vi "RLSET.vi"(8 "错误输入（无错误）":errorcluster, 9 "BIT_L":string, 10 "BIT_H":string) -> (0 "error out":errorcluster caption="错误输出")   [LabVIEW 2018]
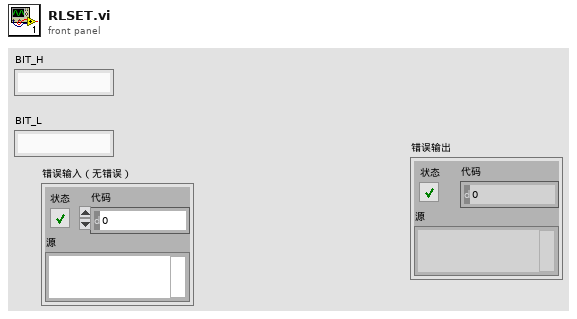
[diagram p1: front panel]
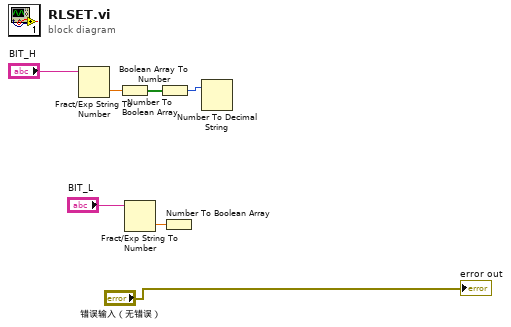
[diagram p0: block diagram]
diagram:
  n1 = Fract/Exp String To Number(string="BIT_H") -> (number=w6:dbl)  [unwired: 3 in, 1 out]
  n2 = Number To Boolean Array(number=w6) -> (Boolean array=w4:bool[])
  n3 = Fract/Exp String To Number(string="BIT_L") -> (number=w5:dbl)  [unwired: 3 in, 1 out]
  n4 = Boolean Array To Number(Boolean array=w4) -> (number=w7:u32)
  n5 = Number To Boolean Array(number=w5) -> ()  [unwired: 1 out]
  n6 = Number To Decimal String(number=w7) -> ()  [unwired: 2 out]
  "error out" <- "错误输入（无错误）"
